vi "Set-display-value.vi"(8 "error in (no error)":errorcluster, 9 "Value":variant, 10 "Display name":T1, 11 "UI ref. in":refnum<data-value>) -> (0 "error out":errorcluster, 3 "UI ref.":refnum<data-value>)   [LabVIEW 2013, in "CameraVision.lvlib" / "CV-UI.lvclass"]
uses:
  CV-UI.lvclass
  Display-names.ctl
  CV-UI.lvclass/CV-UI.ctl
  Read Display refs.vi
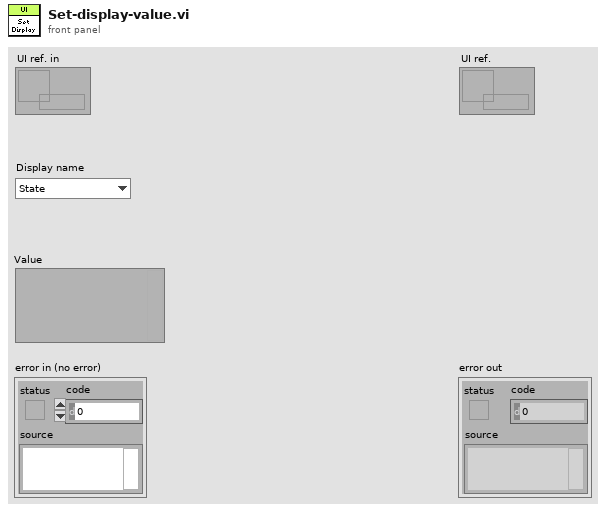
[diagram p1: front panel]
types:
  T1 = typedef "CameraVision.lvlib/CV-UI.lvclass/Display-names.ctl" = enum16{"State", "Action", "Current image", "Framerate", "Frametime", "Process buffer", "Storage buffer", "Free disk space", "Total disk space", "Information", "Histogram", "Camera 1", "Camera 2", "Camera 1 chart", "Camera 2 chart", "Browser", "Temperature", "Map", "Status overview", "Characteristics", "Temper characteristics"}
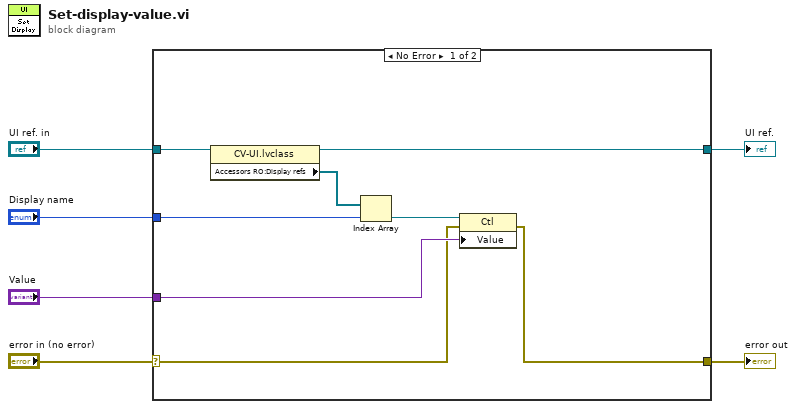
[diagram p0: block diagram]
diagram:
  n1 = case shown="No Error" "error in (no error)" {
    selector: "error in (no error)" -> [w9 w15]
    tunnel: [w8 w15] -> w5
    tunnel: [w7 w16] -> w3
    tunnel: "UI ref. in" -> [w14 w16]
    tunnel: "Display name" -> [w12 _]
    tunnel: "Value" -> [w10 _]
    frame No Error {
      n2 = property class="CV-UI.lvclass"(reference=w14) -> (reference out=w7:refnum<data-value>, "Accessors RO:Display refs"=w13:refnum<vi>[])  [unwired: 1 in, 1 out]
      n3 = Index Array(array=w13, index=w12) -> (element=w11:refnum<vi>)
      n4 = property class="Ctl"(reference=w11, error in=w9, "Value"=w10) -> (error out=w8:errorcluster)  [unwired: 1 out]
    }
    frame Error {
    }
  }
  "error out" <- w5
  "UI ref." <- w3
